vi "TEST - Search Array.vi"(8 "error in (no error)":errorcluster) -> (0 "error out":errorcluster, 2 "Pass?":bool=TRUE)   [LabVIEW 2020]
doc: "This VI template can be used for the functional testing of VIs; this implementation includes handling for the testing of polymorphic VIs, and the polymorphic elements should be removed if not needed.\n\nCoded by Douglas A. Femec, January 24, 2006.\n\nCopyright (c) 2005-2006 MKS Instruments, Inc.\nAll rights reserved."
uses:
  TEST - Search Array - Inputs.ctl
  Polymorphizer+ Data Type.ctl
  TEST - Search Array - Outputs.ctl
  source/library/Search Array/Search 1D Array (EXT).vi
  source/library/Search Array/Search 1D Array (I64).vi
  source/library/Search Array/Search 1D Array (U64).vi
  source/library/Search Array/Search 1D Array (LVObject).vi
  source/library/Search Array/Search 1D Array (DBL).vi
  source/library/Search Array/Search 1D Array (SGL).vi
  source/library/Search Array/Search 1D Array (I32).vi
  source/library/Search Array/Search 1D Array (I16).vi
  source/library/Search Array/Search 1D Array (I8).vi
  source/library/Search Array/Search 1D Array (U32).vi
  source/library/Search Array/Search 1D Array (U16).vi
  source/library/Search Array/Search 1D Array (U8).vi
  source/library/Search Array/Search 1D Array (CXT).vi
  source/library/Search Array/Search 1D Array (CDB).vi
  source/library/Search Array/Search 1D Array (CSG).vi
  source/library/Search Array/Search 1D Array (Boolean).vi
  source/library/Search Array/Search 1D Array (String).vi
  source/library/Search Array/Search 1D Array (Path).vi
  source/library/Search Array/Search 1D Array (Variant).vi
  TestClass/TestClass.lvclass
panel:
  out "Generated Outputs":T1[][](array[typedef])
  in  "Expected Outputs":T1[](array[typedef])=[{"Description"="Expecting no elements found", "Indices of Found Elements"=[]}, {"Description"="Expecting no elements found", "Indices of Found Elements"=[]}, {"Description"="Expecting no elements found", "Indices of Found Elements"=[]}, {"Description"="Expecting no elements found", "Indices of Found Elements"=[]}, {"Description"="Expecting no elements found", "Indices of Found Elements"=[]}, {"Description"="Expecting no elements found", "Indices of Found Elements"=[]}, {"Description"="Expecting one element found", "Indices of Found Elements"=[0]}, {"Description"="Expecting no elements found", "Indices of Found Elements"=[]}, {"Description"="Expecting two elements found", "Indices of Found Elements"=[1, 3]}, {"Description"="Expecting two elements found", "Indices of Found Elements"=[1, 3]}, {"Description"="Expecting two elements found", "Indices of Found Elements"=[0, 2]}, {"Description"="Expecting one element found", "Indices of Found Elements"=[2]}, {"Description"="Expecting one element found", "Indices of Found Elements"=[0]}, {"Description"="Expecting no elements found", "Indices of Found Elements"=[]}, {"Description"="Expecting one element found", "Indices of Found Elements"=[1]}, {"Description"="Expecting one element found", "Indices of Found Elements"=[1]}, {"Description"="Expecting no elements found", "Indices of Found Elements"=[]}, {"Description"="Expecting no elements found", "Indices of Found Elements"=[]}, {"Description"="Expecting four elements found", "Indices of Found Elements"=[0, 1, 2, 3]}, {"Description"="Expecting three elements found", "Indices of Found Elements"=[1, 2, 3]}]
  in  "Inputs":T2[](array[typedef])=[{"Description"="Empty array, looking for 0, starting at 0", "Data Types to Test"=[enum."EXT", enum."DBL", enum."SGL", enum."I32", enum."I16", enum."I8", enum."U32", enum."U16", enum."U8", enum."CXT", enum."CDB", enum."CSG", enum."String", enum."Path", enum."Variant", enum."Boolean", enum."I64", enum."U64", enum."LabVIEW Object"], "Array In"=[], "Element Data"=0.0, "Start Index (0)"=0}, {"Description"="Empty array, looking for 0, starting at 1", "Data Types to Test"=[enum."EXT", enum."DBL", enum."SGL", enum."I32", enum."I16", enum."I8", enum."U32", enum."U16", enum."U8", enum."CXT", enum."CDB", enum."CSG", enum."String", enum."Path", enum."Variant", enum."Boolean", enum."I64", enum."U64", enum."LabVIEW Object"], "Array In"=[], "Element Data"=0.0, "Start Index (0)"=1}, {"Description"="Empty array, looking for 1, starting at 0", "Data Types to Test"=[enum."EXT", enum."DBL", enum."SGL", enum."I32", enum."I16", enum."I8", enum."U32", enum."U16", enum."U8", enum."CXT", enum."CDB", enum."CSG", enum."String", enum."Path", enum."Variant", enum."Boolean", enum."I64", enum."U64", enum."LabVIEW Object"], "Array In"=[], "Element Data"=1.0, "Start Index (0)"=0}, {"Description"="Empty array, looking for 1, starting at 1", "Data Types to Test"=[enum."EXT", enum."DBL", enum."SGL", enum."I32", enum."I16", enum."I8", enum."U32", enum."U16", enum."U8", enum."CXT", enum."CDB", enum."CSG", enum."String", enum."Path", enum."Variant", enum."Boolean", enum."I64", enum."U64", enum."LabVIEW Object"], "Array In"=[], "Element Data"=1.0, "Start Index (0)"=1}, {"Description"="Array with one element, looking for 0, starting at 0", "Data Types to Test"=[enum."EXT", enum."DBL", enum."SGL", enum."I32", enum."I16", enum."I8", enum."U32", enum."U16", enum."U8", enum."CXT", enum."CDB", enum."CSG", enum."String", enum."Path", enum."Variant", enum."Boolean", enum."I64", enum."U64", enum."LabVIEW Object"], "Array In"=[1.0], "Element Data"=0.0, "Start Index (0)"=0}, {"Description"="Array with one element, looking for 0, starting at 1", "Data Types to Test"=[enum."EXT", enum."DBL", enum."SGL", enum."I32", enum."I16", enum."I8", enum."U32", enum."U16", enum."U8", enum."CXT", enum."CDB", enum."CSG", enum."String", enum."Path", enum."Variant", enum."Boolean", enum."I64", enum."U64", enum."LabVIEW Object"], "Array In"=[1.0], "Element Data"=0.0, "Start Index (0)"=1}, {"Description"="Array with one element, looking for 1, starting at 0", "Data Types to Test"=[enum."EXT", enum."DBL", enum."SGL", enum."I32", enum."I16", enum."I8", enum."U32", enum."U16", enum."U8", enum."CXT", enum."CDB", enum."CSG", enum."String", enum."Path", enum."Variant", enum."Boolean", enum."I64", enum."U64", enum."LabVIEW Object"], "Array In"=[1.0], "Element Data"=1.0, "Start Index (0)"=0}, {"Description"="Array with one element, looking for 1, starting at 1", "Data Types to Test"=[enum."EXT", enum."DBL", enum."SGL", enum."I32", enum."I16", enum."I8", enum."U32", enum."U16", enum."U8", enum."CXT", enum."CDB", enum."CSG", enum."String", enum."Path", enum."Variant", enum."Boolean", enum."I64", enum."U64", enum."LabVIEW Object"], "Array In"=[1.0], "Element Data"=1.0, "Start Index (0)"=1}, {"Description"="Array with one each of doubled elements, looking for 0, starting at 0", "Data Types to Test"=[enum."EXT", enum."DBL", enum."SGL", enum."I32", enum."I16", enum."I8", enum."U32", enum."U16", enum."U8", enum."CXT", enum."CDB", enum."CSG", enum."String", enum."Path", enum."Variant", enum."Boolean", enum."I64", enum."U64", enum."LabVIEW Object"], "Array In"=[1.0, 0.0, 1.0, 0.0], "Element Data"=0.0, "Start Index (0)"=0}, {"Description"="Array with one each of doubled elements, looking for 0, starting at 1", "Data Types to Test"=[enum."EXT", enum."DBL", enum."SGL", enum."I32", enum."I16", enum."I8", enum."U32", enum."U16", enum."U8", enum."CXT", enum."CDB", enum."CSG", enum."String", enum."Path", enum."Variant", enum."Boolean", enum."I64", enum."U64", enum."LabVIEW Object"], "Array In"=[1.0, 0.0, 1.0, 0.0], "Element Data"=0.0, "Start Index (0)"=1}, {"Description"="Array with one each of doubled elements, looking for 1, starting at 0", "Data Types to Test"=[enum."EXT", enum."DBL", enum."SGL", enum."I32", enum."I16", enum."I8", enum."U32", enum."U16", enum."U8", enum."CXT", enum."CDB", enum."CSG", enum."String", enum."Path", enum."Variant", enum."Boolean", enum."I64", enum."U64", enum."LabVIEW Object"], "Array In"=[1.0, 0.0, 1.0, 0.0], "Element Data"=1.0, "Start Index (0)"=0}, {"Description"="Array with one each of doubled elements, looking for 1, starting at 1", "Data Types to Test"=[enum."EXT", enum."DBL", enum."SGL", enum."I32", enum."I16", enum."I8", enum."U32", enum."U16", enum."U8", enum."CXT", enum."CDB", enum."CSG", enum."String", enum."Path", enum."Variant", enum."Boolean", enum."I64", enum."U64", enum."LabVIEW Object"], "Array In"=[1.0, 0.0, 1.0, 0.0], "Element Data"=1.0, "Start Index (0)"=1}, {"Description"="Array with one of each element, looking for 0, starting at 0", "Data Types to Test"=[enum."EXT", enum."DBL", enum."SGL", enum."I32", enum."I16", enum."I8", enum."U32", enum."U16", enum."U8", enum."CXT", enum."CDB", enum."CSG", enum."String", enum."Path", enum."Variant", enum."Boolean", enum."I64", enum."U64", enum."LabVIEW Object"], "Array In"=[0.0, 1.0], "Element Data"=0.0, "Start Index (0)"=0}, {"Description"="Array with one of each element, looking for 0, starting at 1", "Data Types to Test"=[enum."EXT", enum."DBL", enum."SGL", enum."I32", enum."I16", enum."I8", enum."U32", enum."U16", enum."U8", enum."CXT", enum."CDB", enum."CSG", enum."String", enum."Path", enum."Variant", enum."Boolean", enum."I64", enum."U64", enum."LabVIEW Object"], "Array In"=[0.0, 1.0], "Element Data"=0.0, "Start Index (0)"=1}, {"Description"="Array with one of each element, looking for 1, starting at 0", "Data Types to Test"=[enum."EXT", enum."DBL", enum."SGL", enum."I32", enum."I16", enum."I8", enum."U32", enum."U16", enum."U8", enum."CXT", enum."CDB", enum."CSG", enum."String", enum."Path", enum."Variant", enum."Boolean", enum."I64", enum."U64", enum."LabVIEW Object"], "Array In"=[0.0, 1.0], "Element Data"=1.0, "Start Index (0)"=0}, {"Description"="Array with one of each element, looking for 1, starting at 1", "Data Types to Test"=[enum."EXT", enum."DBL", enum."SGL", enum."I32", enum."I16", enum."I8", enum."U32", enum."U16", enum."U8", enum."CXT", enum."CDB", enum."CSG", enum."String", enum."Path", enum."Variant", enum."Boolean", enum."I64", enum."U64", enum."LabVIEW Object"], "Array In"=[0.0, 1.0], "Element Data"=1.0, "Start Index (0)"=1}, {"Description"="Array with four of one element, looking for 0, starting at 0", "Data Types to Test"=[enum."EXT", enum."DBL", enum."SGL", enum."I32", enum."I16", enum."I8", enum."U32", enum."U16", enum."U8", enum."CXT", enum."CDB", enum."CSG", enum."String", enum."Path", enum."Variant", enum."Boolean", enum."I64", enum."U64", enum."LabVIEW Object"], "Array In"=[1.0, 1.0, 1.0, 1.0], "Element Data"=0.0, "Start Index (0)"=0}, {"Description"="Array with four of one element, looking for 0, starting at 1", "Data Types to Test"=[enum."EXT", enum."DBL", enum."SGL", enum."I32", enum."I16", enum."I8", enum."U32", enum."U16", enum."U8", enum."CXT", enum."CDB", enum."CSG", enum."String", enum."Path", enum."Variant", enum."Boolean", enum."I64", enum."U64", enum."LabVIEW Object"], "Array In"=[1.0, 1.0, 1.0, 1.0], "Element Data"=0.0, "Start Index (0)"=1}, {"Description"="Array with four of one element, looking for 1, starting at 0", "Data Types to Test"=[enum."EXT", enum."DBL", enum."SGL", enum."I32", enum."I16", enum."I8", enum."U32", enum."U16", enum."U8", enum."CXT", enum."CDB", enum."CSG", enum."String", enum."Path", enum."Variant", enum."Boolean", enum."I64", enum."U64", enum."LabVIEW Object"], "Array In"=[1.0, 1.0, 1.0, 1.0], "Element Data"=1.0, "Start Index (0)"=0}, {"Description"="Array with four of one element, looking for 1, starting at 1", "Data Types to Test"=[enum."EXT", enum."DBL", enum."SGL", enum."I32", enum."I16", enum."I8", enum."U32", enum."U16", enum."U8", enum."CXT", enum."CDB", enum."CSG", enum."String", enum."Path", enum."Variant", enum."Boolean", enum."I64", enum."U64", enum."LabVIEW Object"], "Array In"=[1.0, 1.0, 1.0, 1.0], "Element Data"=1.0, "Start Index (0)"=1}] {"Element Data" format="%.2f"; "Array In" format="%.2f"}
  # "Copyright (c) 2005-2006 MKS Instruments, Inc.\nAll rights reserved."
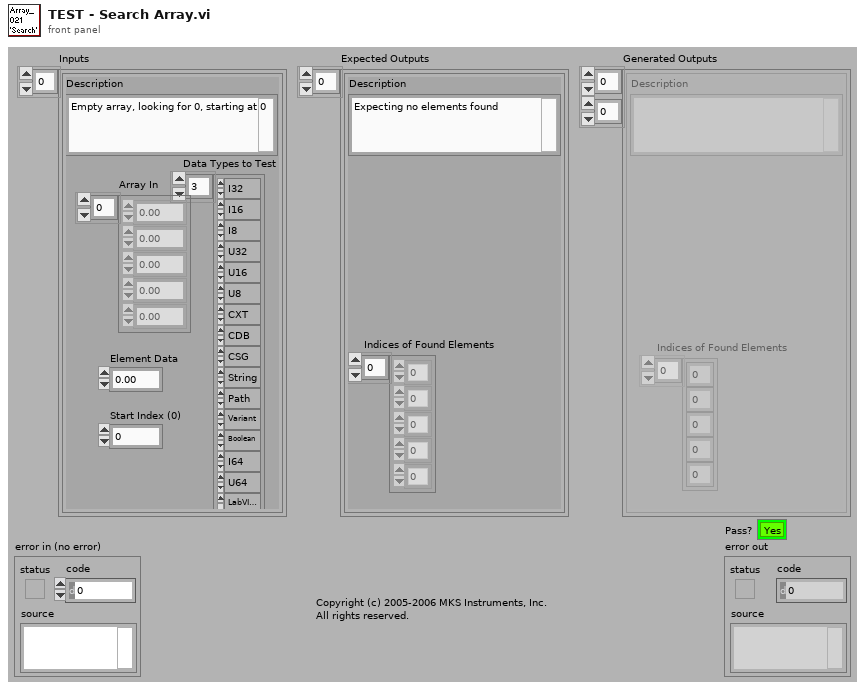
[diagram p1: front panel]
types:
  T1 = typedef "TEST - Search Array - Outputs.ctl" = cluster{"Description":string, "Indices of Found Elements":i32[]}
  T2 = typedef "TEST - Search Array - Inputs.ctl" = cluster{"Description":string, "Data Types to Test":T3[], "Array In":sgl[], "Element Data":sgl, "Start Index (0)":i32}
  T3 = typedef "Polymorphizer+ Data Type.ctl" = enum16{"EXT", "DBL", "SGL", "I32", "I16", "I8", "U32", "U16", "U8", "CXT", "CDB", "CSG", "Boolean", "String", "Path", "Variant", "CTL-REF", "GEN-REF", "GObj-REF", "VI-REF", "ENUM", "ERR", "FILE-REF", "MENU-REF", "MENU-RING", "PICT-RING", "TXT&PICT-RING", "TXT-RING", "I64", "U64", "LabVIEW Object"}
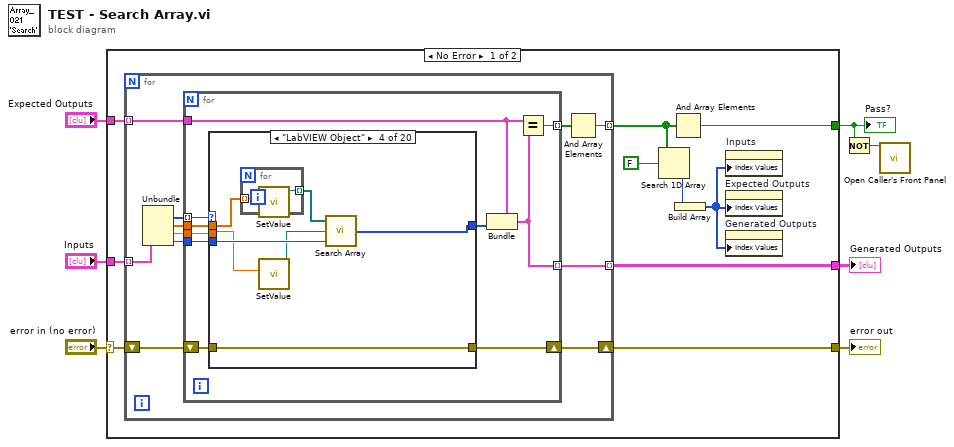
[diagram p0: block diagram]
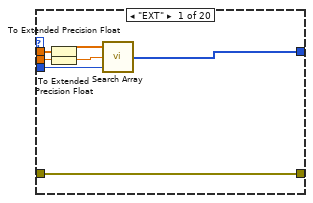
[diagram p2: hidden frame]
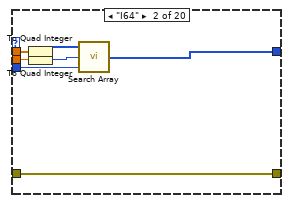
[diagram p3: hidden frame]
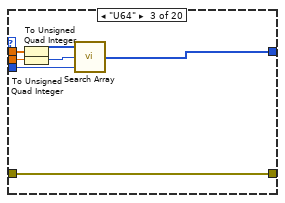
[diagram p4: hidden frame]
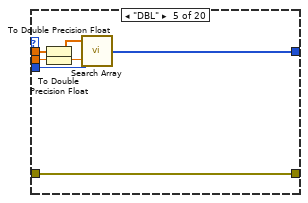
[diagram p5: hidden frame]
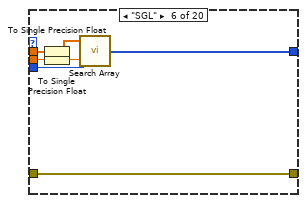
[diagram p6: hidden frame]
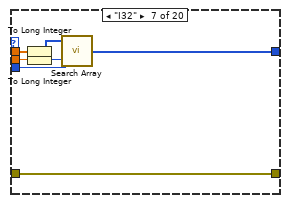
[diagram p7: hidden frame]
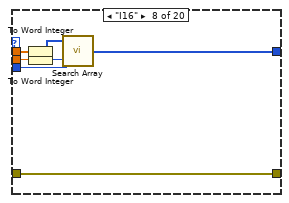
[diagram p8: hidden frame]
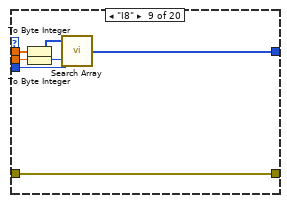
[diagram p9: hidden frame]
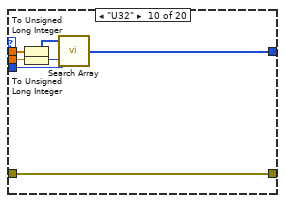
[diagram p10: hidden frame]
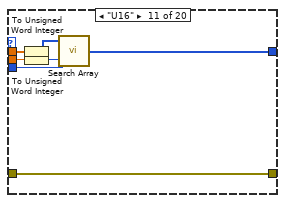
[diagram p11: hidden frame]
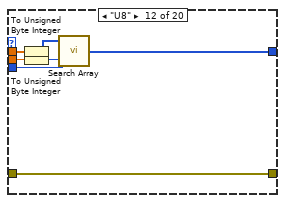
[diagram p12: hidden frame]
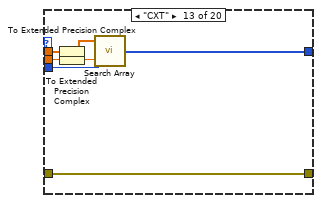
[diagram p13: hidden frame]
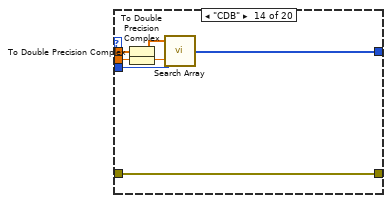
[diagram p14: hidden frame]
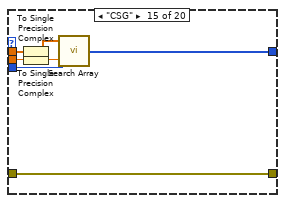
[diagram p15: hidden frame]
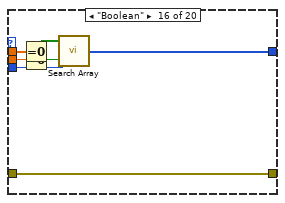
[diagram p16: hidden frame]
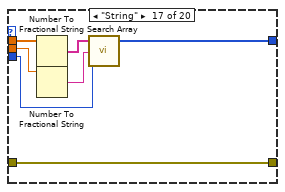
[diagram p17: hidden frame]
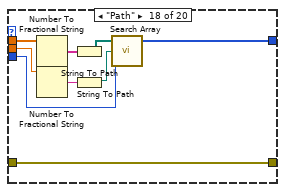
[diagram p18: hidden frame]
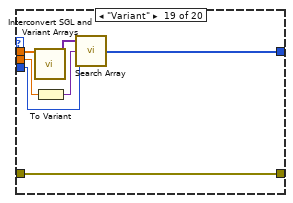
[diagram p19: hidden frame]
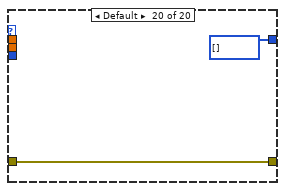
[diagram p20: hidden frame]
diagram:
  n1 = case shown="No Error" "error in (no error)" {
    selector: "error in (no error)" -> [w16 w178]
    tunnel: [w17 w178] -> w6
    tunnel: "Expected Outputs" -> [w14 _]
    tunnel: "Inputs" -> [w15 _]
    tunnel: [w13 _] -> w3
    tunnel: [w12 _] -> w2
    frame No Error {
      n2 = for {
        shift-right: [w23] -> w17
        shift-left: w16 -> [w24]
        tunnel: w15 -> [w25] mode=indexing
        tunnel: w14 -> [w28] mode=indexing
        tunnel: [w27] -> w13 mode=indexing
        tunnel: [w22] -> w11 mode=indexing
        n3 = Unbundle(w25) -> ("Data Types to Test"=w21:T3[], "Array In"=w20:sgl[], "Element Data"=w19:sgl, "Start Index (0)"=w18:i32)  [unwired: 1 out]
        n4 = for {
          tunnel: w28 -> [w38]
          tunnel: [w36] -> w27 mode=indexing
          tunnel: [w37] -> w26 mode=indexing
          shift-right: [w32] -> w23
          shift-left: w24 -> [w33]
          tunnel: w21 -> [w34] mode=indexing
          tunnel: w20 -> [w35]
          tunnel: w19 -> [w30]
          tunnel: w18 -> [w29]
          n5 = case shown="\"LabVIEW Object\"" w34 {
            tunnel: w35 -> [w42 w49 w56 w64 w73 w80 w87 w94 w101 w108 w115 w122 w129 w136 w143 w150 w158 w166 w174 _]
            tunnel: [w44 w51 w58 w60 w74 w81 w88 w95 w102 w109 w116 w123 w130 w137 w144 w151 w156 w164 w172 i32[] [] ("indices of removed elements")] -> w31
            tunnel: w33 -> [w45 w52 w59 w66 w75 w82 w89 w96 w103 w110 w117 w124 w131 w138 w145 w152 w159 w167 w175 w177]
            tunnel: [w45 w52 w59 w66 w75 w82 w89 w96 w103 w110 w117 w124 w131 w138 w145 w152 w159 w167 w175 w177] -> w32
            tunnel: w30 -> [w40 w47 w54 w63 w70 w77 w84 w91 w98 w105 w112 w119 w126 w133 w140 w147 w153 w160 w170 _]
            tunnel: w29 -> [w41 w48 w55 w65 w71 w78 w85 w92 w99 w106 w113 w120 w127 w134 w141 w148 w155 w163 w171 _]
            frame "EXT" {
              n6 = To Extended Precision Float(1:w42) -> (0:w43:ext[])
              n7 = To Extended Precision Float(1:w40) -> (0:w39:ext)
              n8 = call-poly "Search Array.vi"("Array"=w43, "Element Data"=w39, "Start Index (0)"=w41) -> ("Indices of Elements"=w44:i32[])  [unwired: 6 in]
            }
            frame "I64" {
              n9 = To Quad Integer(1:w49) -> (0:w50:i64[])
              n10 = To Quad Integer(1:w47) -> (0:w46:i64)
              n11 = call-poly "Search Array.vi"("Array"=w50, "Element Data"=w46, "Start Index (0)"=w48) -> ("Indices of Elements"=w51:i32[])  [unwired: 6 in]
            }
            frame "U64" {
              n12 = To Unsigned Quad Integer(1:w56) -> (0:w57:u64[])
              n13 = To Unsigned Quad Integer(1:w54) -> (0:w53:u64)
              n14 = call-poly "Search Array.vi"("Array"=w57, "Element Data"=w53, "Start Index (0)"=w55) -> ("Indices of Elements"=w58:i32[])  [unwired: 6 in]
            }
            frame "LabVIEW Object" {
              n15 = for {
                tunnel: w64 -> [w68] mode=indexing
                tunnel: [w67] -> w61 mode=indexing
                n16 = call "SetValue.vi"("Value"=w68) -> ("TestClass out"=w67:refnum<class "TestClass.lvclass">)  [unwired: 9 in, 1 out]
              }
              n17 = call "SetValue.vi"("Value"=w63) -> ("TestClass out"=w62:refnum<class "TestClass.lvclass">)  [unwired: 9 in, 1 out]
              n18 = call-poly "Search Array.vi"("Array"=w61, "Element Data"=w62, "Start Index (0)"=w65) -> ("Indices of Elements"=w60:i32[])  [unwired: 6 in]
            }
            frame "DBL" {
              n19 = To Double Precision Float(number=w73) -> (double precision float=w72:dbl[])
              n20 = To Double Precision Float(number=w70) -> (double precision float=w69:dbl)
              n21 = call-poly "Search Array.vi"("Array"=w72, "Element Data"=w69, "Start Index (0)"=w71) -> ("Indices of Elements"=w74:i32[])  [unwired: 6 in]
            }
            frame "SGL" {
              n22 = To Single Precision Float(number=w80) -> (single precision float=w79:sgl[])
              n23 = To Single Precision Float(number=w77) -> (single precision float=w76:sgl)
              n24 = call-poly "Search Array.vi"("Array"=w79, "Element Data"=w76, "Start Index (0)"=w78) -> ("Indices of Elements"=w81:i32[])  [unwired: 6 in]
            }
            frame "I32" {
              n25 = To Long Integer(number=w87) -> (32bit integer=w86:i32[])
              n26 = To Long Integer(number=w84) -> (32bit integer=w83:i32)
              n27 = call-poly "Search Array.vi"("Array"=w86, "Element Data"=w83, "Start Index (0)"=w85) -> ("Indices of Elements"=w88:i32[])  [unwired: 6 in]
            }
            frame "I16" {
              n28 = To Word Integer(number=w94) -> (16bit integer=w93:i16[])
              n29 = To Word Integer(number=w91) -> (16bit integer=w90:i16)
              n30 = call-poly "Search Array.vi"("Array"=w93, "Element Data"=w90, "Start Index (0)"=w92) -> ("Indices of Elements"=w95:i32[])  [unwired: 6 in]
            }
            frame "I8" {
              n31 = To Byte Integer(number=w101) -> (8bit integer=w100:i8[])
              n32 = To Byte Integer(number=w98) -> (8bit integer=w97:i8)
              n33 = call-poly "Search Array.vi"("Array"=w100, "Element Data"=w97, "Start Index (0)"=w99) -> ("Indices of Elements"=w102:i32[])  [unwired: 6 in]
            }
            frame "U32" {
              n34 = To Unsigned Long Integer(number=w108) -> (unsigned 32bit integer=w107:u32[])
              n35 = To Unsigned Long Integer(number=w105) -> (unsigned 32bit integer=w104:u32)
              n36 = call-poly "Search Array.vi"("Array"=w107, "Element Data"=w104, "Start Index (0)"=w106) -> ("Indices of Elements"=w109:i32[])  [unwired: 6 in]
            }
            frame "U16" {
              n37 = To Unsigned Word Integer(number=w115) -> (unsigned 16bit integer=w114:u16[])
              n38 = To Unsigned Word Integer(number=w112) -> (unsigned 16bit integer=w111:u16)
              n39 = call-poly "Search Array.vi"("Array"=w114, "Element Data"=w111, "Start Index (0)"=w113) -> ("Indices of Elements"=w116:i32[])  [unwired: 6 in]
            }
            frame "U8" {
              n40 = To Unsigned Byte Integer(number=w122) -> (unsigned 8bit integer=w121:u8[])
              n41 = To Unsigned Byte Integer(number=w119) -> (unsigned 8bit integer=w118:u8)
              n42 = call-poly "Search Array.vi"("Array"=w121, "Element Data"=w118, "Start Index (0)"=w120) -> ("Indices of Elements"=w123:i32[])  [unwired: 6 in]
            }
            frame "CXT" {
              n43 = To Extended Precision Complex(1:w129) -> (0:w128:cxt[])
              n44 = To Extended Precision Complex(1:w126) -> (0:w125:cxt)
              n45 = call-poly "Search Array.vi"("Array"=w128, "Element Data"=w125, "Start Index (0)"=w127) -> ("Indices of Elements"=w130:i32[])  [unwired: 6 in]
            }
            frame "CDB" {
              n46 = To Double Precision Complex(1:w136) -> (0:w135:cdb[])
              n47 = To Double Precision Complex(1:w133) -> (0:w132:cdb)
              n48 = call-poly "Search Array.vi"("Array"=w135, "Element Data"=w132, "Start Index (0)"=w134) -> ("Indices of Elements"=w137:i32[])  [unwired: 6 in]
            }
            frame "CSG" {
              n49 = To Single Precision Complex(1:w143) -> (0:w142:csg[])
              n50 = To Single Precision Complex(1:w140) -> (0:w139:csg)
              n51 = call-poly "Search Array.vi"("Array"=w142, "Element Data"=w139, "Start Index (0)"=w141) -> ("Indices of Elements"=w144:i32[])  [unwired: 6 in]
            }
            frame "Boolean" {
              n52 = Equal To 0?(x=w150) -> (x = 0?=w149:bool[])
              n53 = Equal To 0?(x=w147) -> (x = 0?=w146:bool)
              n54 = call-poly "Search Array.vi"("Array"=w149, "Element Data"=w146, "Start Index (0)"=w148) -> ("Indices of Elements"=w151:i32[])  [unwired: 6 in]
            }
            frame "String" {
              n55 = Number To Fractional String(number=w158) -> (F-format string=w157:string[])  [unwired: 3 in]
              n56 = Number To Fractional String(number=w153) -> (F-format string=w154:string)  [unwired: 3 in]
              n57 = call-poly "Search Array.vi"("Array"=w157, "Element Data"=w154, "Start Index (0)"=w155) -> ("Indices of Elements"=w156:i32[])  [unwired: 6 in]
            }
            frame "Path" {
              n58 = Number To Fractional String(number=w166) -> (F-format string=w168:string[])  [unwired: 3 in]
              n59 = Number To Fractional String(number=w160) -> (F-format string=w162:string)  [unwired: 3 in]
              n60 = String To Path(string=w168) -> (path=w165:path[])
              n61 = String To Path(string=w162) -> (path=w161:path)
              n62 = call-poly "Search Array.vi"("Array"=w165, "Element Data"=w161, "Start Index (0)"=w163) -> ("Indices of Elements"=w164:i32[])  [unwired: 6 in]
            }
            frame "Variant" {
              n63 = call "Interconvert SGL and Variant Arrays.vi"("SGL 1D Array In"=w174) -> ("Variant 1D Array Out"=w173:variant[])  [unwired: 10 in, 4 out]
              n64 = To Variant(anything=w170) -> (Variant=w169:variant)
              n65 = call-poly "Search Array.vi"("Array"=w173, "Element Data"=w169, "Start Index (0)"=w171) -> ("Indices of Elements"=w172:i32[])  [unwired: 6 in]
            }
            frame Default {
            }
          }
          n66 = Bundle(cluster=w38, "Indices of Found Elements"=w31) -> (w36:T1)  [unwired: 1 in]
          n67 = Equal?(x=w38, y=w36) -> (x = y?=w37:bool)
        }
        n68 = And Array Elements(Boolean array=w26) -> (logical AND=w22:bool)
      }
      n69 = Search 1D Array(1D array=w11, element=FALSE) -> (index of element=w9:i32)  [unwired: 1 in]
      n70 = And Array Elements(Boolean array=w11) -> (logical AND=w12:bool)
      n71 = Build Array(w9) -> (w8:i32[])
      n72 = property on="Inputs" class="Arr (strict)"("Index Values"=w8) -> ()  [unwired: 2 in, 2 out]
      n73 = property on="Expected Outputs" class="Arr (strict)"("Index Values"=w8) -> ()  [unwired: 2 in, 2 out]
      n74 = property on="Generated Outputs" class="Arr (strict)"("Index Values"=w8) -> ()  [unwired: 2 in, 2 out]
    }
    frame Error {
    }
  }
  "error out" <- w6
  "Pass?" <- w2
  "Generated Outputs" <- w3
  n75 = Not(x=w2) -> (.not. x?=w1:bool)
  n76 = call "Open Caller's Front Panel.vi"("Open?"=w1) -> ()  [unwired: 14 in, 1 out]
